vi "UpdateMetricCacheHighRate.vi"(8 "error in (no error)":errorcluster, 9 "HighRate":bool, 10 "metric definition instance id":string, 11 "metric cache in":variant) -> (0 "error out":errorcluster, 3 "metric cache out":variant)   [LabVIEW 2017, in "AnalysisHelper.lvlib"]
uses:
  <vilib>/addons/InsightCM/Utilities/Analysis/Shared/AnalysisHelper.lvlib
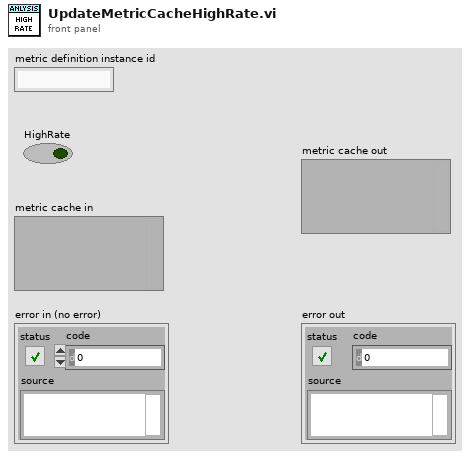
[diagram p1: front panel]
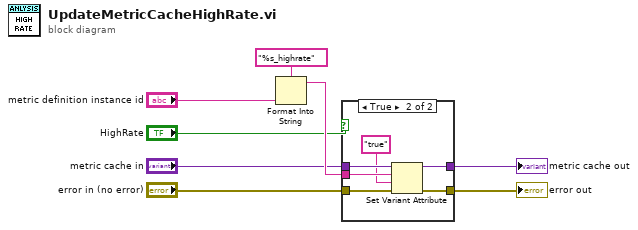
[diagram p0: block diagram]
diagram:
  n1 = Format Into String(format string="%s_highrate", "metric definition instance id") -> (resulting string=w8:string)  [unwired: 2 in, 1 out]
  n2 = case shown="True" "HighRate" {
    tunnel: "metric cache in" -> [w10 w16]
    tunnel: [w10 w15] -> w2
    tunnel: "error in (no error)" -> [w9 w14]
    tunnel: [w9 w13] -> w3
    tunnel: w8 -> [_ w12]
    frame False {
    }
    frame True {
      n3 = Set Variant Attribute(Variant=w16, name=w12, value="true" ("format string"), error in=w14) -> (Variant out=w15:variant, error out=w13:errorcluster)  [unwired: 1 out]
    }
  }
  "error out" <- w3
  "metric cache out" <- w2
